vi "ROI grp-UI manage disabled states.vi"(8 "error in (no error)":errorcluster, 9 "UI elemente enabled?":T1(ring)) -> (0 "error out":errorcluster)   [LabVIEW 2020]
uses:
  Globals/gl_ROI grp window globals.vi
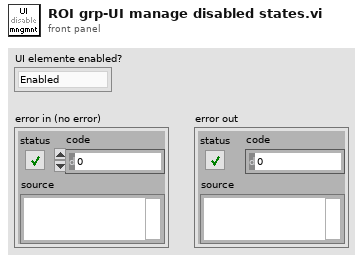
[diagram p1: front panel]
types:
  T1 = enum8{"Enabled", "Disabled", "Disabled and Grayed Out"}
  T2 = typedef "ROI grp-window ctrl refs.ctl" = cluster{"This VI":refnum<vi>, "Pane":refnum<vi>, "Table":refnum<vi>}
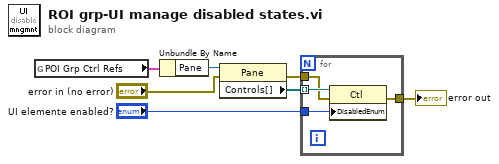
[diagram p0: block diagram]
diagram:
  n1 = global read "gl_ROI grp window globals.vi" "POI Grp Ctrl Refs"() -> (w1:T2)
  n2 = Unbundle By Name(w1) -> ("Pane"=w7:refnum<vi>)
  n3 = property on="Property Node" class="Pane"(reference=w7, error in="error in (no error)") -> (error out=w2:errorcluster, "Controls[]"=w6:refnum<vi>[])  [unwired: 1 out]
  n4 = for {
    tunnel: w6 -> [w11] mode=indexing
    tunnel: "UI elemente enabled?" -> [w10]
    tunnel: [w9] -> w4
    tunnel: w2 -> [w8]
    n5 = property on="Property Node" class="Ctl"(reference=w11, error in=w8, "DisabledEnum"=w10) -> (error out=w9:errorcluster)  [unwired: 1 out]
  }
  "error out" <- w4
